vi "GetUIs.vi"(11 "AllVIs":refnum<vi>[](array[refnum])) -> (3 "TAFProjDocumentType:FrontPanelGUIOut":refnum<class "FrontPanelGUI.lvclass">)   [LabVIEW 2021, in "TAF Proj Document Type.lvlib" / "Project Parser.lvlib"]
uses:
  <vilib>/Wovalab/AntiDoc/Document Type/Add-ons/LabVIEW TAF Project/Project Parser/Project Parser.lvlib
  <vilib>/Wovalab/AntiDoc/Document Type/Add-ons/LabVIEW TAF Project/FrontPanelGUI/FrontPanelGUI.lvclass
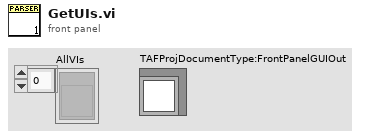
[diagram p1: front panel]
types:
  T1 = typedef "LVBookmarkInfoTypeDef.ctl" = cluster{"Bookmark Reference":u32, "Bookmark Tag":string, "Label Text":string}[]
  T2 = typedef "imagedata.ctl" = cluster{"image type":i32, "image depth":i32, "image":u8[], "mask":u8[], "colors":u32[], "Rectangle":cluster{"left":i16, "top":i16, "right":i16, "bottom":i16}}
  T3 = cluster{"VI Name":string, "Lib Name":string, "Controls":string[], "ControlImage":T2[], "Descriptions":string[]}
  T4 = cluster{"VI Name":string, "Lib Name":string, "Controls":string[], "ControlImage":T2[], "Descriptions":string[]}[]
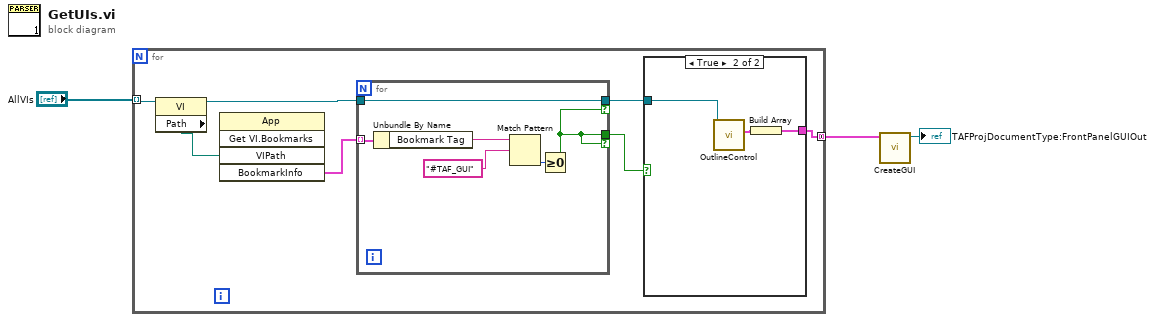
[diagram p0: block diagram]
diagram:
  n1 = for {
    tunnel: "AllVIs" -> [w7] mode=indexing
    tunnel: [w9] -> w2 mode=concatenating
    n2 = property class="VI"(reference=w7) -> (reference out=w4:refnum<vi>, "Path"=w6:path)  [unwired: 1 in, 1 out]
    n3 = invoke class="App" method="Get VI.Bookmarks"("VIPath"=w6) -> ("BookmarkInfo"=w5:T1)  [unwired: 4 in, 4 out]
    n4 = for {
      tunnel: w5 -> [w19] mode=indexing
      tunnel: [w16] -> w10 if=w14
      tunnel: w4 -> [w16]
      tunnel: [w14] -> w8 if=w14
      n5 = Unbundle By Name(w19) -> ("Bookmark Tag"=w18:string)
      n6 = Match Pattern(string=w18, regular expression="#TAF_GUI") -> (offset past match=w15:i32)  [unwired: 1 in, 3 out]
      n7 = Greater Or Equal To 0?(x=w15) -> (x >= 0?=w14:bool)
    }
    n8 = case shown="True" w8 {
      tunnel: w10 -> [_ w13]
      tunnel: [_ w11] -> w9
      frame False {
      }
      frame True {
        n9 = call <vilib>:"OutlineControl.vi"("ViReference"=w13) -> ("Images"=w12:T3)  [unwired: 10 in]
        n10 = Build Array(w12) -> (w11:T4)
      }
    }
  }
  n11 = call <vilib>:"CreateGUI.vi"("GUIs"=w2) -> ("TAFProjDocumentType:FrontPanelGUIOut"=→"TAFProjDocumentType:FrontPanelGUIOut":refnum<class "FrontPanelGUI.lvclass">)  [unwired: 9 in, 1 out]
